vi "WriteGroup.vi"(7 "LabVIEW Web Service Request":refnum<class "Web Request.lvclass">, 10 "groupName":T2, 11 "groupData":T1) -> ()   [LabVIEW 2013]
uses:
  <vilib>/wsapi/Web Request.lvclass
  <vilib>/NI/TagWebClient/API/String Controls/groupName.ctl
  <vilib>/NI/TagWebClient/API/String Controls/groupData.ctl
  <vilib>/NI/TagWebClient/API/tagweb client API.lvlib
  <vilib>/NI/Tag Bus/tag/Data Type.ctl
  <vilib>/NI/Tag Bus/tag/tag descriptor.lvclass
  <vilib>/NI/Tag Bus/table/allocation specification.ctl
  <vilib>/NI/Tag Bus/table/data table.lvlib
panel:
  # "Use the Web Service Request input terminal to call the VIs on the Web Services palette. Do not remove it from the connector pane unless you don't need access to the palette."
  # "Each additional control wired to the connector pane will be available as an input in the URL. To include an indicator in terminal-mode output (the default setting), it must also be wired to the connector pane."
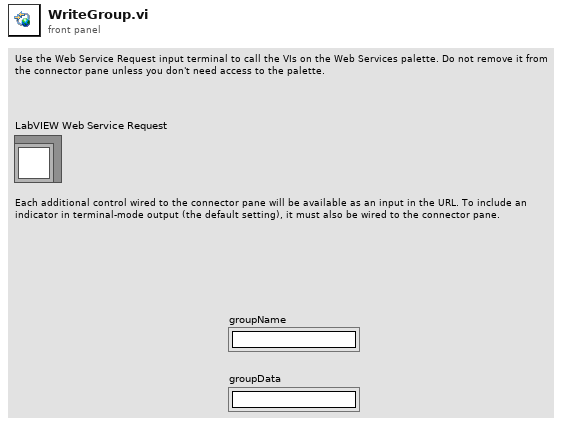
[diagram p1: front panel]
types:
  T1 = typedef "tagweb client API.lvlib/groupData.ctl" = string
  T2 = typedef "tagweb client API.lvlib/groupName.ctl" = string
  T3 = typedef "tag bus.lvlib/data table.lvlib/allocation specification.ctl" = cluster{"data type":T4, "size":i32}
  T4 = typedef "tag bus.lvlib/tag descriptor.lvclass/Data Type.ctl" = enum16{"Double", "Single", "I64", "I32", "I16", "I8", "U64", "U32", "U16", "U8", "Boolean", "String", "Array of Double", "Array of Single", "Array of I64", "Array of I32", "Array of I16", "Array of I8", "Array of U64", "Array of U32", "Array of U16", "Array of U8", "Array of Boolean", "Array of String"}
  T5 = typedef "tag bus.lvlib/data table.lvlib/data table.ctl" = cluster{"Double":dbl[], "Single":sgl[], "I64":i64[], "I32":i32[], "I16":i16[], "I8":i8[], "U64":u64[], "U32":u32[], "U16":u16[], "U8":u8[], "Boolean":bool[], "String":string[], "Array of Double":cluster{"DBL Array":dbl[]}[], "Array of Single":cluster{"SGL Array":sgl[]}[], "Array of I64":cluster{"I64 Array":i64[]}[], "Array of I32":cluster{"I32 Array":i32[]}[], "Array of I16":cluster{"I16 Array":i16[]}[], "Array of I8":cluster{"I8 Array":i8[]}[], "Array of U64":cluster{"U64 Array":u64[]}[], "Array of U32":cluster{"U32 Array":u32[]}[], "Array of U16":cluster{"U16 Array":u16[]}[], "Array of U8":cluster{"U8 Array":u8[]}[], "Array of Boolean":cluster{"Boolean Array":bool[]}[], "Array of String":cluster{"String Array":string[]}[]}
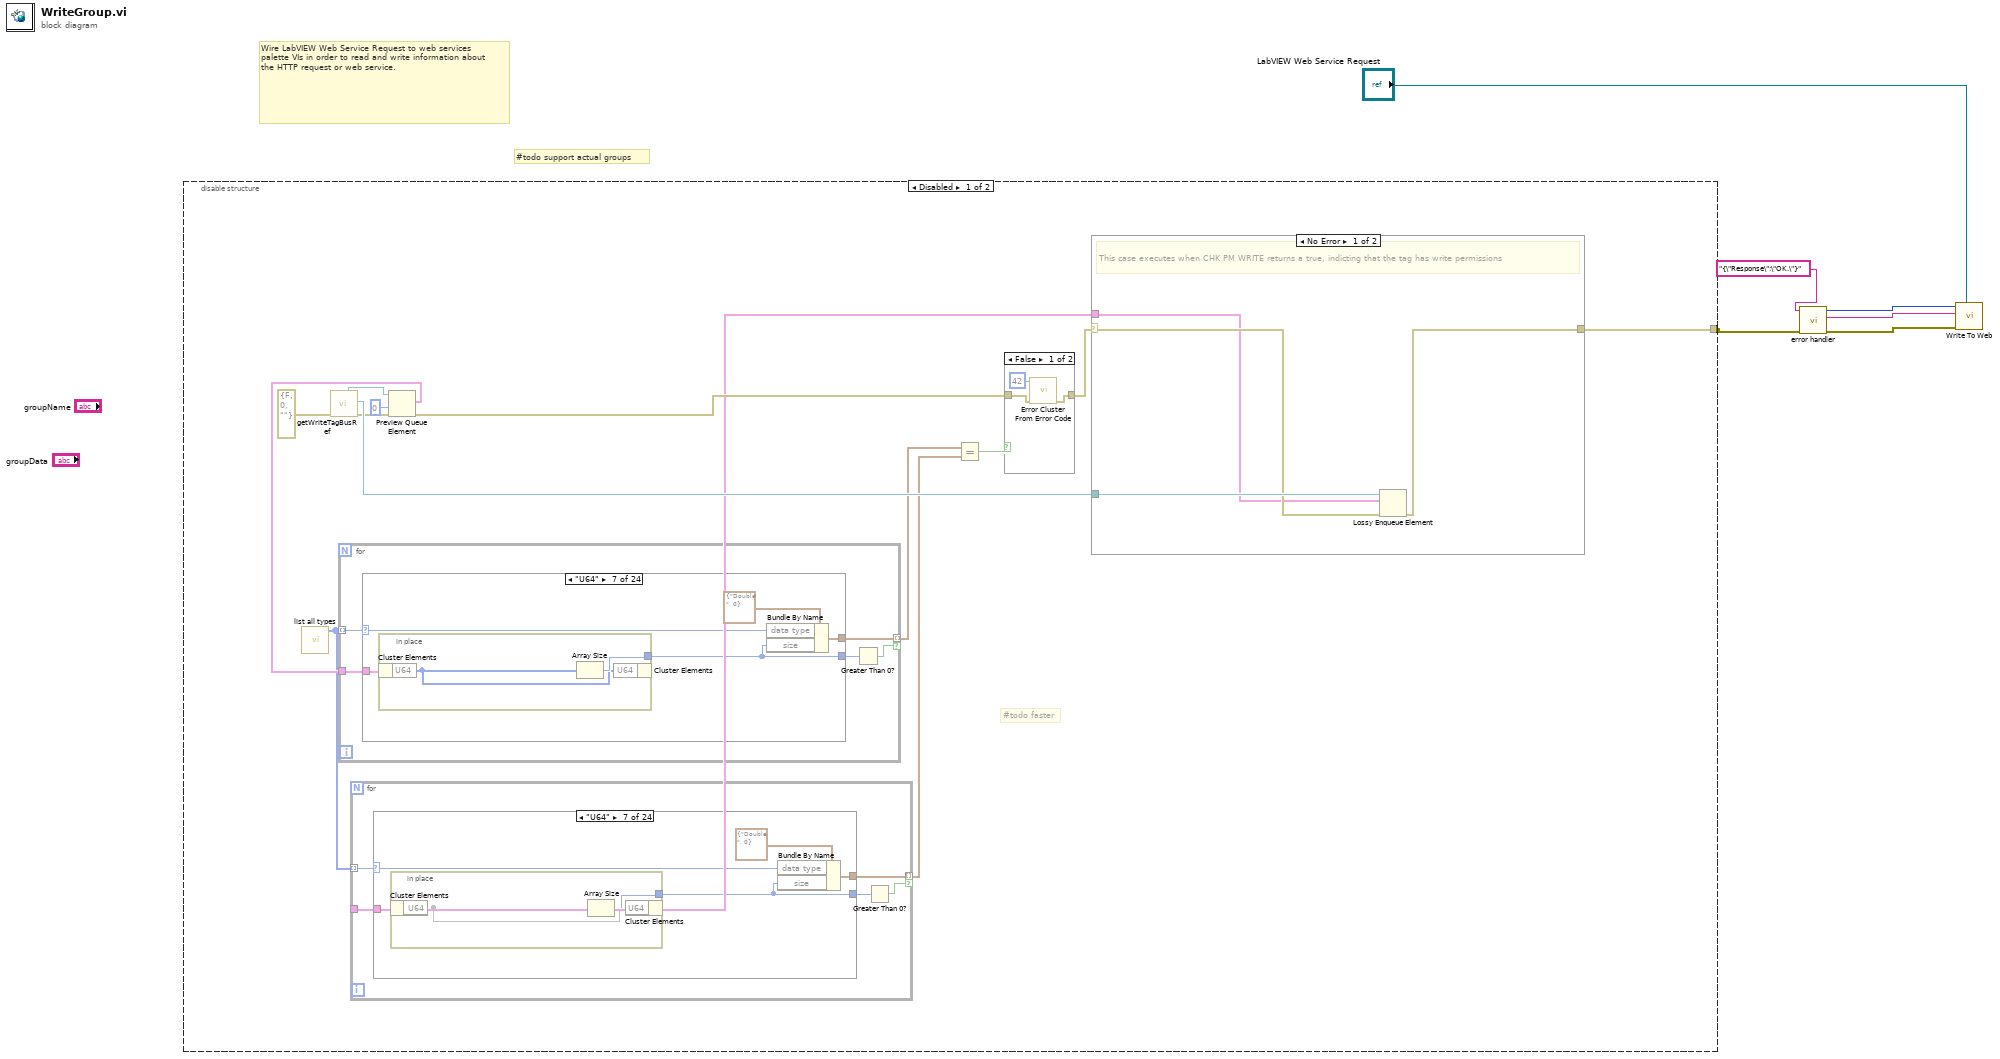
[diagram p0: block diagram]
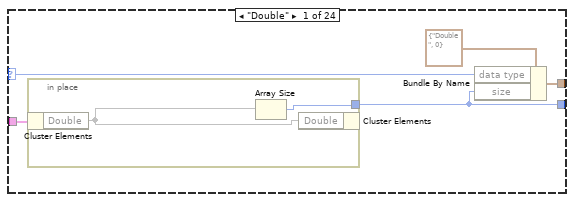
[diagram p3: hidden frame]
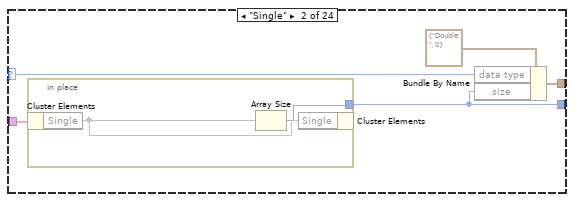
[diagram p4: hidden frame]
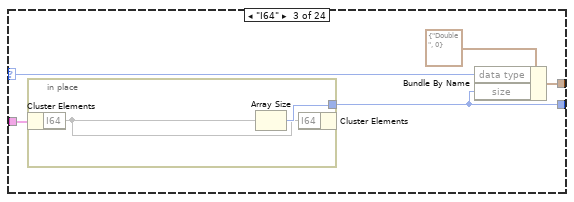
[diagram p5: hidden frame]
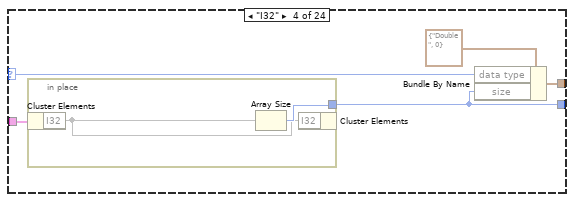
[diagram p6: hidden frame]
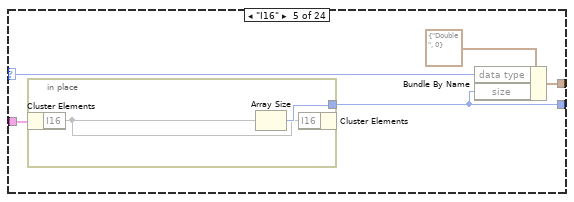
[diagram p7: hidden frame]
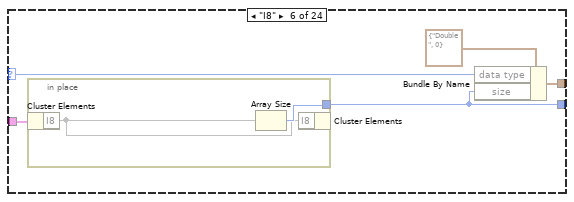
[diagram p8: hidden frame]
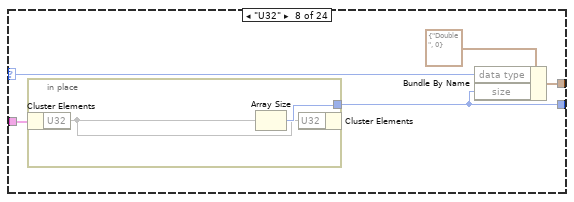
[diagram p9: hidden frame]
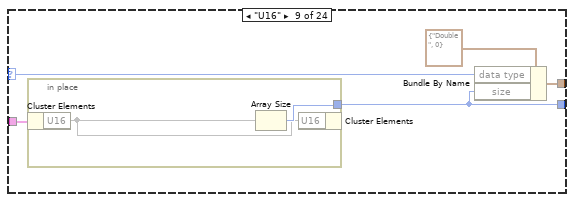
[diagram p10: hidden frame]
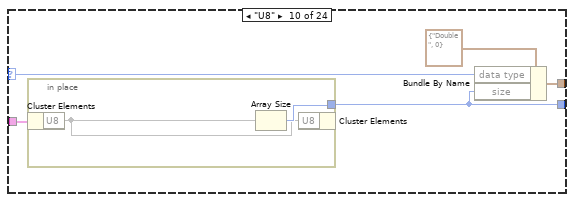
[diagram p11: hidden frame]
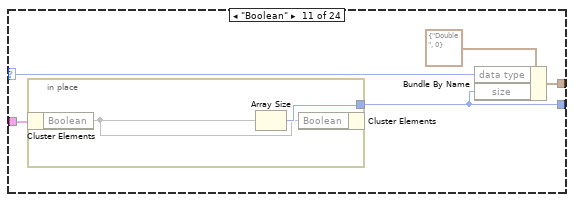
[diagram p12: hidden frame]
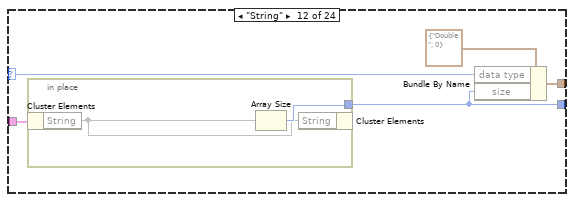
[diagram p13: hidden frame]
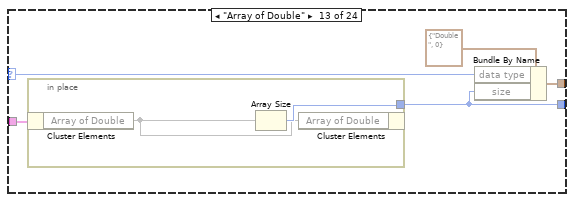
[diagram p14: hidden frame]
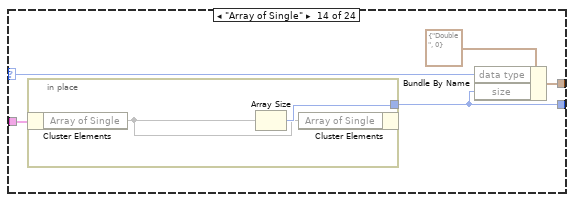
[diagram p15: hidden frame]
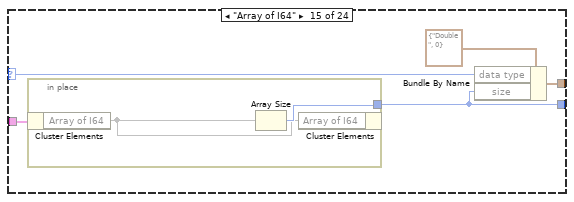
[diagram p16: hidden frame]
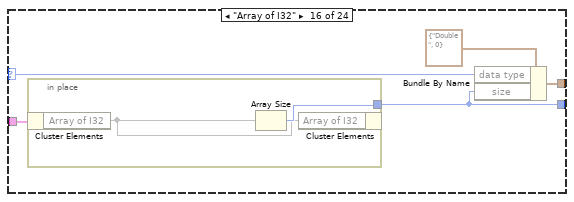
[diagram p17: hidden frame]
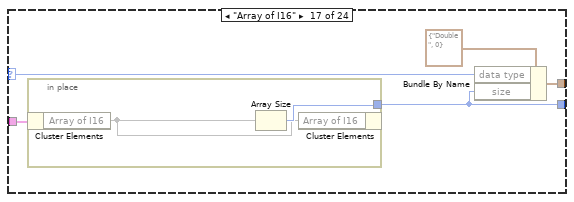
[diagram p18: hidden frame]
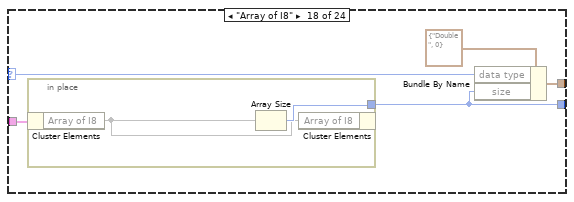
[diagram p19: hidden frame]
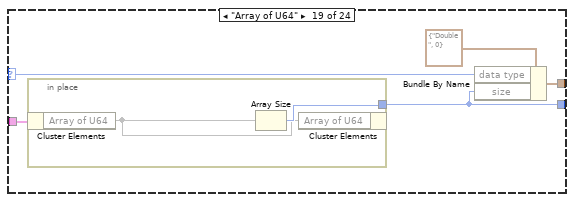
[diagram p20: hidden frame]
diagram:
  # "#todo support actual groups"
  # "Wire LabVIEW Web Service Request to web services palette VIs in order to read and write information about the HTTP request or web service."
  n1 = disable-structure shown="Disabled" {
    disable-tunnel: [w20 _] -> w6
    frame Disabled {
      # "#todo faster"
      n2 = call <vilib>:"list all types.vi"() -> ("all types"=w13:T4[])  [unwired: 11 in]
      n3 = call "getWriteTagBusRef.vi"("error in"=errorcluster {"status"=FALSE, "code"=0, "source"=""} ("error in (no error)")) -> ("error out"=w17:errorcluster, "write tx data table"=w18:refnum<queue>, "actual write data table"=w15:refnum<queue>)  [unwired: 6 in, 2 out]
      n4 = Preview Queue Element(queue=w15, timeout in ms (-1)=0, error in (no error)=w17) -> (element=w14:T5, error out=w16:errorcluster)  [unwired: 2 out]
      n5 = for {
        tunnel: w13 -> [w202] mode=indexing
        tunnel: [w200] -> w10 mode=indexing if=w199
        tunnel: w14 -> [w201]
        n6 = case shown="\"U64\"" w202 {
          selector: w202 -> [w205 w212 w219 w226 w233 w240 w247 w254 w261 w268 w275 w282 w289 w296 w303 w310 w317 w324 w331 w338 w345 w352 w359 w366]
          tunnel: w201 -> [w207 w214 w221 w228 w235 w242 w249 w256 w263 w270 w277 w284 w291 w298 w305 w312 w319 w326 w333 w340 w347 w354 w361 w368]
          tunnel: [w204 w211 w218 w225 w232 w239 w246 w253 w260 w267 w274 w281 w288 w295 w302 w309 w316 w323 w330 w337 w344 w351 w358 w365] -> w200
          tunnel: [w203 w210 w217 w224 w231 w238 w245 w252 w259 w266 w273 w280 w287 w294 w301 w308 w315 w322 w329 w336 w343 w350 w357 w364] -> w198
          frame "Double" {
            n7 = in-place {
              in-place-border: [w209] -> w203
              n8 = in-place-cluster #1(w207) -> ("Double"=w208:dbl[])
              n9 = Array Size(array=w208) -> (size(s)=w209:i32)
              n10 = in-place-cluster #1("Double"=w208) -> ()  [unwired: 1 out]
            }
            n11 = Bundle By Name(cluster=T3 {"data type"=enum."Double", "size"=0} ("allocation"), "data type"=w205, "size"=w203) -> (w204:T3)
          }
          frame "Single" {
            n12 = in-place {
              in-place-border: [w216] -> w210
              n13 = in-place-cluster #2(w214) -> ("Single"=w215:sgl[])
              n14 = Array Size(array=w215) -> (size(s)=w216:i32)
              n15 = in-place-cluster #2("Single"=w215) -> ()  [unwired: 1 out]
            }
            n16 = Bundle By Name(cluster=T3 {"data type"=enum."Double", "size"=0} ("allocation"), "data type"=w212, "size"=w210) -> (w211:T3)
          }
          frame "I64" {
            n17 = in-place {
              in-place-border: [w223] -> w217
              n18 = in-place-cluster #3(w221) -> ("I64"=w222:i64[])
              n19 = Array Size(array=w222) -> (size(s)=w223:i32)
              n20 = in-place-cluster #3("I64"=w222) -> ()  [unwired: 1 out]
            }
            n21 = Bundle By Name(cluster=T3 {"data type"=enum."Double", "size"=0} ("allocation"), "data type"=w219, "size"=w217) -> (w218:T3)
          }
          frame "I32" {
            n22 = in-place {
              in-place-border: [w230] -> w224
              n23 = in-place-cluster #4(w228) -> ("I32"=w229:i32[])
              n24 = Array Size(array=w229) -> (size(s)=w230:i32)
              n25 = in-place-cluster #4("I32"=w229) -> ()  [unwired: 1 out]
            }
            n26 = Bundle By Name(cluster=T3 {"data type"=enum."Double", "size"=0} ("allocation"), "data type"=w226, "size"=w224) -> (w225:T3)
          }
          frame "I16" {
            n27 = in-place {
              in-place-border: [w237] -> w231
              n28 = in-place-cluster #5(w235) -> ("I16"=w236:i16[])
              n29 = Array Size(array=w236) -> (size(s)=w237:i32)
              n30 = in-place-cluster #5("I16"=w236) -> ()  [unwired: 1 out]
            }
            n31 = Bundle By Name(cluster=T3 {"data type"=enum."Double", "size"=0} ("allocation"), "data type"=w233, "size"=w231) -> (w232:T3)
          }
          frame "I8" {
            n32 = in-place {
              in-place-border: [w244] -> w238
              n33 = in-place-cluster #6(w242) -> ("I8"=w243:i8[])
              n34 = Array Size(array=w243) -> (size(s)=w244:i32)
              n35 = in-place-cluster #6("I8"=w243) -> ()  [unwired: 1 out]
            }
            n36 = Bundle By Name(cluster=T3 {"data type"=enum."Double", "size"=0} ("allocation"), "data type"=w240, "size"=w238) -> (w239:T3)
          }
          frame "U64" {
            n37 = in-place {
              in-place-border: [w251] -> w245
              n38 = in-place-cluster #7(w249) -> ("U64"=w250:u64[])
              n39 = Array Size(array=w250) -> (size(s)=w251:i32)
              n40 = in-place-cluster #7("U64"=w250) -> ()  [unwired: 1 out]
            }
            n41 = Bundle By Name(cluster=T3 {"data type"=enum."Double", "size"=0} ("allocation"), "data type"=w247, "size"=w245) -> (w246:T3)
          }
          frame "U32" {
            n42 = in-place {
              in-place-border: [w258] -> w252
              n43 = in-place-cluster #8(w256) -> ("U32"=w257:u32[])
              n44 = Array Size(array=w257) -> (size(s)=w258:i32)
              n45 = in-place-cluster #8("U32"=w257) -> ()  [unwired: 1 out]
            }
            n46 = Bundle By Name(cluster=T3 {"data type"=enum."Double", "size"=0} ("allocation"), "data type"=w254, "size"=w252) -> (w253:T3)
          }
          frame "U16" {
            n47 = in-place {
              in-place-border: [w265] -> w259
              n48 = in-place-cluster #9(w263) -> ("U16"=w264:u16[])
              n49 = Array Size(array=w264) -> (size(s)=w265:i32)
              n50 = in-place-cluster #9("U16"=w264) -> ()  [unwired: 1 out]
            }
            n51 = Bundle By Name(cluster=T3 {"data type"=enum."Double", "size"=0} ("allocation"), "data type"=w261, "size"=w259) -> (w260:T3)
          }
          frame "U8" {
            n52 = in-place {
              in-place-border: [w272] -> w266
              n53 = in-place-cluster #10(w270) -> ("U8"=w271:u8[])
              n54 = Array Size(array=w271) -> (size(s)=w272:i32)
              n55 = in-place-cluster #10("U8"=w271) -> ()  [unwired: 1 out]
            }
            n56 = Bundle By Name(cluster=T3 {"data type"=enum."Double", "size"=0} ("allocation"), "data type"=w268, "size"=w266) -> (w267:T3)
          }
          frame "Boolean" {
            n57 = in-place {
              in-place-border: [w279] -> w273
              n58 = in-place-cluster #11(w277) -> ("Boolean"=w278:bool[])
              n59 = Array Size(array=w278) -> (size(s)=w279:i32)
              n60 = in-place-cluster #11("Boolean"=w278) -> ()  [unwired: 1 out]
            }
            n61 = Bundle By Name(cluster=T3 {"data type"=enum."Double", "size"=0} ("allocation"), "data type"=w275, "size"=w273) -> (w274:T3)
          }
          frame "String" {
            n62 = in-place {
              in-place-border: [w286] -> w280
              n63 = in-place-cluster #12(w284) -> ("String"=w285:string[])
              n64 = Array Size(array=w285) -> (size(s)=w286:i32)
              n65 = in-place-cluster #12("String"=w285) -> ()  [unwired: 1 out]
            }
            n66 = Bundle By Name(cluster=T3 {"data type"=enum."Double", "size"=0} ("allocation"), "data type"=w282, "size"=w280) -> (w281:T3)
          }
          frame "Array of Double" {
            n67 = in-place {
              in-place-border: [w293] -> w287
              n68 = in-place-cluster #13(w291) -> ("Array of Double"=w292:cluster{"DBL Array":dbl[]}[])
              n69 = Array Size(array=w292) -> (size(s)=w293:i32)
              n70 = in-place-cluster #13("Array of Double"=w292) -> ()  [unwired: 1 out]
            }
            n71 = Bundle By Name(cluster=T3 {"data type"=enum."Double", "size"=0} ("allocation"), "data type"=w289, "size"=w287) -> (w288:T3)
          }
          frame "Array of Single" {
            n72 = in-place {
              in-place-border: [w300] -> w294
              n73 = in-place-cluster #14(w298) -> ("Array of Single"=w299:cluster{"SGL Array":sgl[]}[])
              n74 = Array Size(array=w299) -> (size(s)=w300:i32)
              n75 = in-place-cluster #14("Array of Single"=w299) -> ()  [unwired: 1 out]
            }
            n76 = Bundle By Name(cluster=T3 {"data type"=enum."Double", "size"=0} ("allocation"), "data type"=w296, "size"=w294) -> (w295:T3)
          }
          frame "Array of I64" {
            n77 = in-place {
              in-place-border: [w307] -> w301
              n78 = in-place-cluster #15(w305) -> ("Array of I64"=w306:cluster{"I64 Array":i64[]}[])
              n79 = Array Size(array=w306) -> (size(s)=w307:i32)
              n80 = in-place-cluster #15("Array of I64"=w306) -> ()  [unwired: 1 out]
            }
            n81 = Bundle By Name(cluster=T3 {"data type"=enum."Double", "size"=0} ("allocation"), "data type"=w303, "size"=w301) -> (w302:T3)
          }
          frame "Array of I32" {
            n82 = in-place {
              in-place-border: [w314] -> w308
              n83 = in-place-cluster #16(w312) -> ("Array of I32"=w313:cluster{"I32 Array":i32[]}[])
              n84 = Array Size(array=w313) -> (size(s)=w314:i32)
              n85 = in-place-cluster #16("Array of I32"=w313) -> ()  [unwired: 1 out]
            }
            n86 = Bundle By Name(cluster=T3 {"data type"=enum."Double", "size"=0} ("allocation"), "data type"=w310, "size"=w308) -> (w309:T3)
          }
          frame "Array of I16" {
            n87 = in-place {
              in-place-border: [w321] -> w315
              n88 = in-place-cluster #17(w319) -> ("Array of I16"=w320:cluster{"I16 Array":i16[]}[])
              n89 = Array Size(array=w320) -> (size(s)=w321:i32)
              n90 = in-place-cluster #17("Array of I16"=w320) -> ()  [unwired: 1 out]
            }
            n91 = Bundle By Name(cluster=T3 {"data type"=enum."Double", "size"=0} ("allocation"), "data type"=w317, "size"=w315) -> (w316:T3)
          }
          frame "Array of I8" {
            n92 = in-place {
              in-place-border: [w328] -> w322
              n93 = in-place-cluster #18(w326) -> ("Array of I8"=w327:cluster{"I8 Array":i8[]}[])
              n94 = Array Size(array=w327) -> (size(s)=w328:i32)
              n95 = in-place-cluster #18("Array of I8"=w327) -> ()  [unwired: 1 out]
            }
            n96 = Bundle By Name(cluster=T3 {"data type"=enum."Double", "size"=0} ("allocation"), "data type"=w324, "size"=w322) -> (w323:T3)
          }
          frame "Array of U64" {
            n97 = in-place {
              in-place-border: [w335] -> w329
              n98 = in-place-cluster #19(w333) -> ("Array of U64"=w334:cluster{"U64 Array":u64[]}[])
              n99 = Array Size(array=w334) -> (size(s)=w335:i32)
              n100 = in-place-cluster #19("Array of U64"=w334) -> ()  [unwired: 1 out]
            }
            n101 = Bundle By Name(cluster=T3 {"data type"=enum."Double", "size"=0} ("allocation"), "data type"=w331, "size"=w329) -> (w330:T3)
          }
          frame "Array of U32" {
            n102 = in-place {
              in-place-border: [w342] -> w336
              n103 = in-place-cluster #20(w340) -> ("Array of U32"=w341:cluster{"U32 Array":u32[]}[])
              n104 = Array Size(array=w341) -> (size(s)=w342:i32)
              n105 = in-place-cluster #20("Array of U32"=w341) -> ()  [unwired: 1 out]
            }
            n106 = Bundle By Name(cluster=T3 {"data type"=enum."Double", "size"=0} ("allocation"), "data type"=w338, "size"=w336) -> (w337:T3)
          }
          frame "Array of U16" {
            n107 = in-place {
              in-place-border: [w349] -> w343
              n108 = in-place-cluster #21(w347) -> ("Array of U16"=w348:cluster{"U16 Array":u16[]}[])
              n109 = Array Size(array=w348) -> (size(s)=w349:i32)
              n110 = in-place-cluster #21("Array of U16"=w348) -> ()  [unwired: 1 out]
            }
            n111 = Bundle By Name(cluster=T3 {"data type"=enum."Double", "size"=0} ("allocation"), "data type"=w345, "size"=w343) -> (w344:T3)
          }
          frame "Array of U8" {
            n112 = in-place {
              in-place-border: [w356] -> w350
              n113 = in-place-cluster #22(w354) -> ("Array of U8"=w355:cluster{"U8 Array":u8[]}[])
              n114 = Array Size(array=w355) -> (size(s)=w356:i32)
              n115 = in-place-cluster #22("Array of U8"=w355) -> ()  [unwired: 1 out]
            }
            n116 = Bundle By Name(cluster=T3 {"data type"=enum."Double", "size"=0} ("allocation"), "data type"=w352, "size"=w350) -> (w351:T3)
          }
          frame "Array of Boolean" {
            n117 = in-place {
              in-place-border: [w363] -> w357
              n118 = in-place-cluster #23(w361) -> ("Array of Boolean"=w362:cluster{"Boolean Array":bool[]}[])
              n119 = Array Size(array=w362) -> (size(s)=w363:i32)
              n120 = in-place-cluster #23("Array of Boolean"=w362) -> ()  [unwired: 1 out]
            }
            n121 = Bundle By Name(cluster=T3 {"data type"=enum."Double", "size"=0} ("allocation"), "data type"=w359, "size"=w357) -> (w358:T3)
          }
          frame "Array of String" {
            n122 = in-place {
              in-place-border: [w370] -> w364
              n123 = in-place-cluster #24(w368) -> ("Array of String"=w369:cluster{"String Array":string[]}[])
              n124 = Array Size(array=w369) -> (size(s)=w370:i32)
              n125 = in-place-cluster #24("Array of String"=w369) -> ()  [unwired: 1 out]
            }
            n126 = Bundle By Name(cluster=T3 {"data type"=enum."Double", "size"=0} ("allocation"), "data type"=w366, "size"=w364) -> (w365:T3)
          }
        }
        n127 = Greater Than 0?(x=w198) -> (x > 0?=w199:bool)
      }
      n128 = for {
        tunnel: w13 -> [w29] mode=indexing
        tunnel: [w27] -> w11 mode=indexing if=w26
        tunnel: w12 -> [w28]
        n129 = case shown="\"U64\"" w29 {
          selector: w29 -> [w32 w39 w46 w53 w60 w67 w74 w81 w88 w95 w102 w109 w116 w123 w130 w137 w144 w151 w158 w165 w172 w179 w186 w193]
          tunnel: w28 -> [w34 w41 w48 w55 w62 w69 w76 w83 w90 w97 w104 w111 w118 w125 w132 w139 w146 w153 w160 w167 w174 w181 w188 w195]
          tunnel: [w31 w38 w45 w52 w59 w66 w73 w80 w87 w94 w101 w108 w115 w122 w129 w136 w143 w150 w157 w164 w171 w178 w185 w192] -> w27
          tunnel: [w30 w37 w44 w51 w58 w65 w72 w79 w86 w93 w100 w107 w114 w121 w128 w135 w142 w149 w156 w163 w170 w177 w184 w191] -> w25
          frame "Double" {
            n130 = in-place {
              in-place-border: [w36] -> w30
              n131 = in-place-cluster #25(w34) -> ("Double"=w35)
              n132 = Array Size(array=w35) -> (size(s)=w36:i32)
              n133 = in-place-cluster #25("Double"=w35) -> ()  [unwired: 1 out]
            }
            n134 = Bundle By Name(cluster=T3 {"data type"=enum."Double", "size"=0} ("allocation"), "data type"=w32, "size"=w30) -> (w31:T3)
          }
          frame "Single" {
            n135 = in-place {
              in-place-border: [w43] -> w37
              n136 = in-place-cluster #26(w41) -> ("Single"=w42)
              n137 = Array Size(array=w42) -> (size(s)=w43:i32)
              n138 = in-place-cluster #26("Single"=w42) -> ()  [unwired: 1 out]
            }
            n139 = Bundle By Name(cluster=T3 {"data type"=enum."Double", "size"=0} ("allocation"), "data type"=w39, "size"=w37) -> (w38:T3)
          }
          frame "I64" {
            n140 = in-place {
              in-place-border: [w50] -> w44
              n141 = in-place-cluster #27(w48) -> ("I64"=w49)
              n142 = Array Size(array=w49) -> (size(s)=w50:i32)
              n143 = in-place-cluster #27("I64"=w49) -> ()  [unwired: 1 out]
            }
            n144 = Bundle By Name(cluster=T3 {"data type"=enum."Double", "size"=0} ("allocation"), "data type"=w46, "size"=w44) -> (w45:T3)
          }
          frame "I32" {
            n145 = in-place {
              in-place-border: [w57] -> w51
              n146 = in-place-cluster #28(w55) -> ("I32"=w56)
              n147 = Array Size(array=w56) -> (size(s)=w57:i32)
              n148 = in-place-cluster #28("I32"=w56) -> ()  [unwired: 1 out]
            }
            n149 = Bundle By Name(cluster=T3 {"data type"=enum."Double", "size"=0} ("allocation"), "data type"=w53, "size"=w51) -> (w52:T3)
          }
          frame "I16" {
            n150 = in-place {
              in-place-border: [w64] -> w58
              n151 = in-place-cluster #29(w62) -> ("I16"=w63)
              n152 = Array Size(array=w63) -> (size(s)=w64:i32)
              n153 = in-place-cluster #29("I16"=w63) -> ()  [unwired: 1 out]
            }
            n154 = Bundle By Name(cluster=T3 {"data type"=enum."Double", "size"=0} ("allocation"), "data type"=w60, "size"=w58) -> (w59:T3)
          }
          frame "I8" {
            n155 = in-place {
              in-place-border: [w71] -> w65
              n156 = in-place-cluster #30(w69) -> ("I8"=w70)
              n157 = Array Size(array=w70) -> (size(s)=w71:i32)
              n158 = in-place-cluster #30("I8"=w70) -> ()  [unwired: 1 out]
            }
            n159 = Bundle By Name(cluster=T3 {"data type"=enum."Double", "size"=0} ("allocation"), "data type"=w67, "size"=w65) -> (w66:T3)
          }
          frame "U64" {
            n160 = in-place {
              in-place-border: [w78] -> w72
              n161 = in-place-cluster #31(w76) -> ("U64"=w77)
              n162 = Array Size(array=w77) -> (size(s)=w78:i32)
              n163 = in-place-cluster #31("U64"=w77) -> ()  [unwired: 1 out]
            }
            n164 = Bundle By Name(cluster=T3 {"data type"=enum."Double", "size"=0} ("allocation"), "data type"=w74, "size"=w72) -> (w73:T3)
          }
          frame "U32" {
            n165 = in-place {
              in-place-border: [w85] -> w79
              n166 = in-place-cluster #32(w83) -> ("U32"=w84)
              n167 = Array Size(array=w84) -> (size(s)=w85:i32)
              n168 = in-place-cluster #32("U32"=w84) -> ()  [unwired: 1 out]
            }
            n169 = Bundle By Name(cluster=T3 {"data type"=enum."Double", "size"=0} ("allocation"), "data type"=w81, "size"=w79) -> (w80:T3)
          }
          frame "U16" {
            n170 = in-place {
              in-place-border: [w92] -> w86
              n171 = in-place-cluster #33(w90) -> ("U16"=w91)
              n172 = Array Size(array=w91) -> (size(s)=w92:i32)
              n173 = in-place-cluster #33("U16"=w91) -> ()  [unwired: 1 out]
            }
            n174 = Bundle By Name(cluster=T3 {"data type"=enum."Double", "size"=0} ("allocation"), "data type"=w88, "size"=w86) -> (w87:T3)
          }
          frame "U8" {
            n175 = in-place {
              in-place-border: [w99] -> w93
              n176 = in-place-cluster #34(w97) -> ("U8"=w98)
              n177 = Array Size(array=w98) -> (size(s)=w99:i32)
              n178 = in-place-cluster #34("U8"=w98) -> ()  [unwired: 1 out]
            }
            n179 = Bundle By Name(cluster=T3 {"data type"=enum."Double", "size"=0} ("allocation"), "data type"=w95, "size"=w93) -> (w94:T3)
          }
          frame "Boolean" {
            n180 = in-place {
              in-place-border: [w106] -> w100
              n181 = in-place-cluster #35(w104) -> ("Boolean"=w105)
              n182 = Array Size(array=w105) -> (size(s)=w106:i32)
              n183 = in-place-cluster #35("Boolean"=w105) -> ()  [unwired: 1 out]
            }
            n184 = Bundle By Name(cluster=T3 {"data type"=enum."Double", "size"=0} ("allocation"), "data type"=w102, "size"=w100) -> (w101:T3)
          }
          frame "String" {
            n185 = in-place {
              in-place-border: [w113] -> w107
              n186 = in-place-cluster #36(w111) -> ("String"=w112)
              n187 = Array Size(array=w112) -> (size(s)=w113:i32)
              n188 = in-place-cluster #36("String"=w112) -> ()  [unwired: 1 out]
            }
            n189 = Bundle By Name(cluster=T3 {"data type"=enum."Double", "size"=0} ("allocation"), "data type"=w109, "size"=w107) -> (w108:T3)
          }
          frame "Array of Double" {
            n190 = in-place {
              in-place-border: [w120] -> w114
              n191 = in-place-cluster #37(w118) -> ("Array of Double"=w119)
              n192 = Array Size(array=w119) -> (size(s)=w120:i32)
              n193 = in-place-cluster #37("Array of Double"=w119) -> ()  [unwired: 1 out]
            }
            n194 = Bundle By Name(cluster=T3 {"data type"=enum."Double", "size"=0} ("allocation"), "data type"=w116, "size"=w114) -> (w115:T3)
          }
          frame "Array of Single" {
            n195 = in-place {
              in-place-border: [w127] -> w121
              n196 = in-place-cluster #38(w125) -> ("Array of Single"=w126)
              n197 = Array Size(array=w126) -> (size(s)=w127:i32)
              n198 = in-place-cluster #38("Array of Single"=w126) -> ()  [unwired: 1 out]
            }
            n199 = Bundle By Name(cluster=T3 {"data type"=enum."Double", "size"=0} ("allocation"), "data type"=w123, "size"=w121) -> (w122:T3)
          }
          frame "Array of I64" {
            n200 = in-place {
              in-place-border: [w134] -> w128
              n201 = in-place-cluster #39(w132) -> ("Array of I64"=w133)
              n202 = Array Size(array=w133) -> (size(s)=w134:i32)
              n203 = in-place-cluster #39("Array of I64"=w133) -> ()  [unwired: 1 out]
            }
            n204 = Bundle By Name(cluster=T3 {"data type"=enum."Double", "size"=0} ("allocation"), "data type"=w130, "size"=w128) -> (w129:T3)
          }
          frame "Array of I32" {
            n205 = in-place {
              in-place-border: [w141] -> w135
              n206 = in-place-cluster #40(w139) -> ("Array of I32"=w140)
              n207 = Array Size(array=w140) -> (size(s)=w141:i32)
              n208 = in-place-cluster #40("Array of I32"=w140) -> ()  [unwired: 1 out]
            }
            n209 = Bundle By Name(cluster=T3 {"data type"=enum."Double", "size"=0} ("allocation"), "data type"=w137, "size"=w135) -> (w136:T3)
          }
          frame "Array of I16" {
            n210 = in-place {
              in-place-border: [w148] -> w142
              n211 = in-place-cluster #41(w146) -> ("Array of I16"=w147)
              n212 = Array Size(array=w147) -> (size(s)=w148:i32)
              n213 = in-place-cluster #41("Array of I16"=w147) -> ()  [unwired: 1 out]
            }
            n214 = Bundle By Name(cluster=T3 {"data type"=enum."Double", "size"=0} ("allocation"), "data type"=w144, "size"=w142) -> (w143:T3)
          }
          frame "Array of I8" {
            n215 = in-place {
              in-place-border: [w155] -> w149
              n216 = in-place-cluster #42(w153) -> ("Array of I8"=w154)
              n217 = Array Size(array=w154) -> (size(s)=w155:i32)
              n218 = in-place-cluster #42("Array of I8"=w154) -> ()  [unwired: 1 out]
            }
            n219 = Bundle By Name(cluster=T3 {"data type"=enum."Double", "size"=0} ("allocation"), "data type"=w151, "size"=w149) -> (w150:T3)
          }
          frame "Array of U64" {
            n220 = in-place {
              in-place-border: [w162] -> w156
              n221 = in-place-cluster #43(w160) -> ("Array of U64"=w161)
              n222 = Array Size(array=w161) -> (size(s)=w162:i32)
              n223 = in-place-cluster #43("Array of U64"=w161) -> ()  [unwired: 1 out]
            }
            n224 = Bundle By Name(cluster=T3 {"data type"=enum."Double", "size"=0} ("allocation"), "data type"=w158, "size"=w156) -> (w157:T3)
          }
          frame "Array of U32" {
            n225 = in-place {
              in-place-border: [w169] -> w163
              n226 = in-place-cluster #44(w167) -> ("Array of U32"=w168)
              n227 = Array Size(array=w168) -> (size(s)=w169:i32)
              n228 = in-place-cluster #44("Array of U32"=w168) -> ()  [unwired: 1 out]
            }
            n229 = Bundle By Name(cluster=T3 {"data type"=enum."Double", "size"=0} ("allocation"), "data type"=w165, "size"=w163) -> (w164:T3)
          }
          frame "Array of U16" {
            n230 = in-place {
              in-place-border: [w176] -> w170
              n231 = in-place-cluster #45(w174) -> ("Array of U16"=w175)
              n232 = Array Size(array=w175) -> (size(s)=w176:i32)
              n233 = in-place-cluster #45("Array of U16"=w175) -> ()  [unwired: 1 out]
            }
            n234 = Bundle By Name(cluster=T3 {"data type"=enum."Double", "size"=0} ("allocation"), "data type"=w172, "size"=w170) -> (w171:T3)
          }
          frame "Array of U8" {
            n235 = in-place {
              in-place-border: [w183] -> w177
              n236 = in-place-cluster #46(w181) -> ("Array of U8"=w182)
              n237 = Array Size(array=w182) -> (size(s)=w183:i32)
              n238 = in-place-cluster #46("Array of U8"=w182) -> ()  [unwired: 1 out]
            }
            n239 = Bundle By Name(cluster=T3 {"data type"=enum."Double", "size"=0} ("allocation"), "data type"=w179, "size"=w177) -> (w178:T3)
          }
          frame "Array of Boolean" {
            n240 = in-place {
              in-place-border: [w190] -> w184
              n241 = in-place-cluster #47(w188) -> ("Array of Boolean"=w189)
              n242 = Array Size(array=w189) -> (size(s)=w190:i32)
              n243 = in-place-cluster #47("Array of Boolean"=w189) -> ()  [unwired: 1 out]
            }
            n244 = Bundle By Name(cluster=T3 {"data type"=enum."Double", "size"=0} ("allocation"), "data type"=w186, "size"=w184) -> (w185:T3)
          }
          frame "Array of String" {
            n245 = in-place {
              in-place-border: [w197] -> w191
              n246 = in-place-cluster #48(w195) -> ("Array of String"=w196)
              n247 = Array Size(array=w196) -> (size(s)=w197:i32)
              n248 = in-place-cluster #48("Array of String"=w196) -> ()  [unwired: 1 out]
            }
            n249 = Bundle By Name(cluster=T3 {"data type"=enum."Double", "size"=0} ("allocation"), "data type"=w193, "size"=w191) -> (w192:T3)
          }
        }
        n250 = Greater Than 0?(x=w25) -> (x > 0?=w26:bool)
      }
      n251 = Equal?(x=w10, y=w11) -> (x = y?=w9:bool)
      n252 = case shown="False" w9 {
        tunnel: [w22 w24] -> w8
        tunnel: w16 -> [w23 w24]
        frame False {
          n253 = call <vilib>:"Error Cluster From Error Code.vi"("error in (no error)"=w23, "error code (0)"=42) -> ("error out"=w22:errorcluster)  [unwired: 7 in]
        }
        frame True {
        }
      }
      n254 = case shown="No Error" w8 {
        selector: w8 -> [w372 w375]
        tunnel: [w373 w375] -> w20
        tunnel: w18 -> [w374 _]
        tunnel: [w371 _] -> w12
        frame No Error {
          # "This case executes when CHK PM WRITE returns a true, indicting that the tag has write permissions"
          n255 = Lossy Enqueue Element(queue=w374, element=w371, error in (no error)=w372) -> (error out=w373:errorcluster)  [unwired: 3 out]
        }
        frame Error {
          # "This case executes when CHK PM WRITE returns a false, indicating that the tag does not have write permissions"
        }
      }
    }
    frame Enabled {
    }
  }
  n256 = call "error handler.vi"("error in (no error)"=w6, "Success Message"="{\"Response\":\"OK.\"}" ("response string")) -> ("error out"=w4:errorcluster, "Response String"=w2:string, "Response Code"=w3:i32)  [unwired: 7 in]
  n257 = call <vilib>:"Write To Web.vi"("Web Request in"="LabVIEW Web Service Request", "error in (no error)"=w4, "Response String"=w2, "Response Code"=w3) -> ()  [unwired: 7 in, 1 out]
